vi "Read IO_Dir and IO_Rd.vi"(8 "error in (no error)":errorcluster) -> (0 "error out":errorcluster, 2 "IO_Wr":u32, 3 "IO_Dir":u32)   [LabVIEW 2016]
uses:
  Host/Typedefs/IO Buffer Operation.ctl
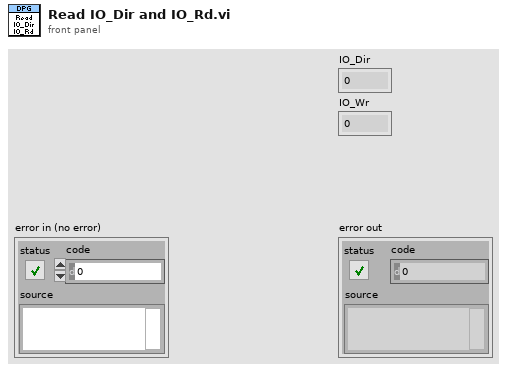
[diagram p1: front panel]
types:
  T1 = typedef "IO Buffer Operation.ctl" = enum16{"Initialize", "Write IO Data_Rd", "Read IO Data_Rd", "Write IO Data_Wr", "Read IO Data_Wr", "Write  IO Data_Dir", "Read  IO Data_Dir", "Write Host to Target FIFO", "Read Host to Target FIFO", "Write Target to Host FIFO", "Read Target to Host FIFO", "Write Monitor Enable?", "Read Monitor Enable?", "Close"}
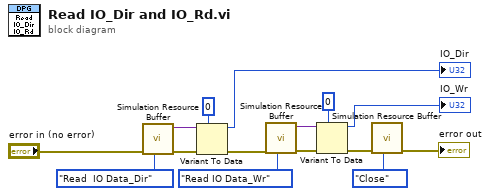
[diagram p0: block diagram]
diagram:
  n1 = call "Simulation Resource Buffer.vi"("IO Buffer Operation"=IO_Buffer_Operation."Read  IO Data_Dir", "error in (no error)"="error in (no error)") -> ("error out"=w10:errorcluster, "Data out"=w9:variant)  [unwired: 7 in, 1 out]
  n2 = Variant To Data(error in=w10, type=u32 0, Variant=w9) -> (data=→"IO_Dir":u32, error out=w8:errorcluster)
  n3 = call "Simulation Resource Buffer.vi"("IO Buffer Operation"=IO_Buffer_Operation."Read IO Data_Wr", "error in (no error)"=w8) -> ("error out"=w7:errorcluster, "Data out"=w6:variant)  [unwired: 7 in, 1 out]
  n4 = Variant To Data(error in=w7, type=u32 0, Variant=w6) -> (data=→"IO_Wr":u32, error out=w5:errorcluster)
  n5 = call "Simulation Resource Buffer.vi"("IO Buffer Operation"=IO_Buffer_Operation."Close", "error in (no error)"=w5) -> ("error out"=→"error out":errorcluster)  [unwired: 7 in, 2 out]
